vi "example.vi"() -> ()   [LabVIEW 2020]
uses:
  g_industrial_cam/Device Enumeration.ctl
  g_industrial_cam/Camera/Camera.lvclass/Camera.ctl
  g_industrial_cam/Buffer/Buffer.lvclass/Buffer.ctl
  g_industrial_cam/Camera/GetSetPixelFormat.vi
  g_industrial_cam/Buffer/Create from Handle.vi
  g_industrial_cam/Camera/Check Not Disconnected.vi
  <vilib>/Utility/error.llb/Error Cluster From Error Code.vi
  g_industrial_cam/Buffer/Buffer.lvclass
  g_industrial_cam/Camera/Camera.lvclass
panel:
  out "error out":errorcluster
  out "Image":T1(plugin-control)
  out "Devices":T2[](array[typedef])
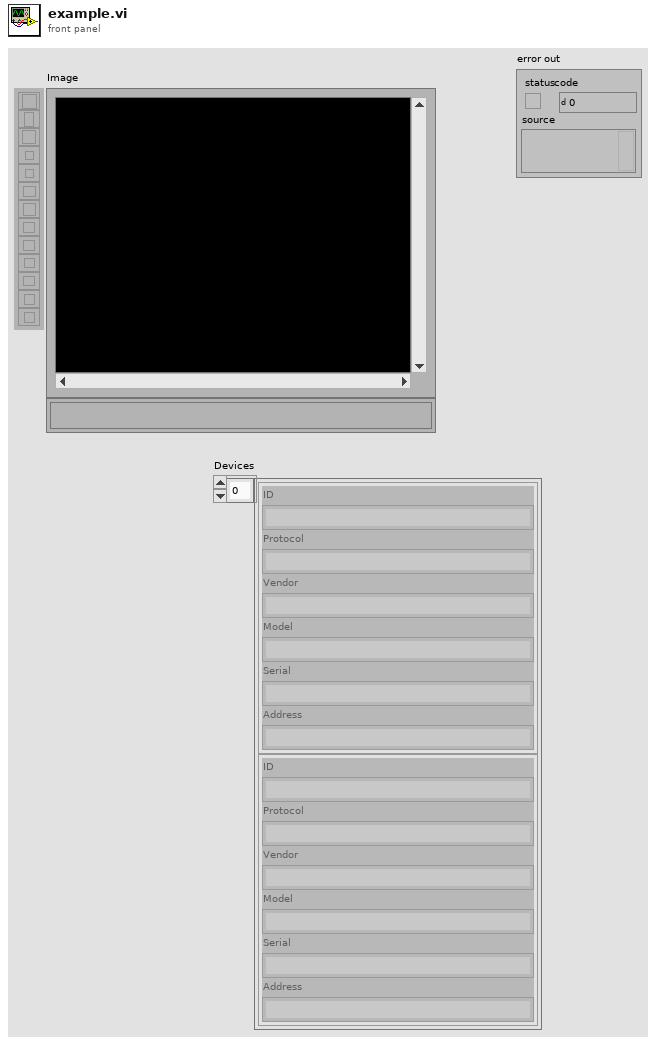
[diagram p1: front panel]
types:
  T1 = typedef "IMAQ Image.ctl" = refnum<image>
  T2 = typedef "Device Enumeration.ctl" = cluster{"ID":string, "Protocol":string, "Vendor":string, "Model":string, "Serial":string, "Address":string}
  T3 = typedef "Image Type" = u32
  T4 = typedef "Buffer.lvclass/Image Size.ctl" = cluster{"Width":u16, "Height":u16}
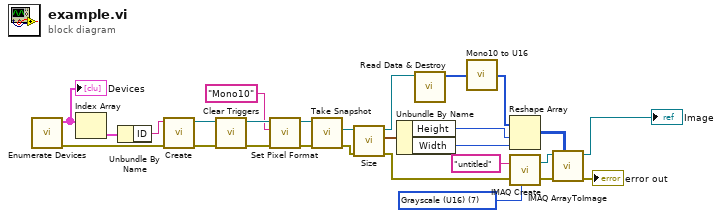
[diagram p0: block diagram]
diagram:
  w27 = T3 7 items=["Grayscale (U8)", "Grayscale (I16)", "Grayscale (SGL)", "Complex (CSG)", "RGB (U32)", "HSL (U32)", "RGB (U64)", "Grayscale (U16)"] ("Image Type")
  n1 = call "Enumerate Devices.vi"() -> ("error out"=w24:errorcluster, "Devices"=w26:T2[])  [unwired: 10 in]
  "Devices" <- w26
  n2 = Index Array(array=w26) -> (element=w25:T2)  [unwired: 1 in]
  n3 = Unbundle By Name(w25) -> ("ID"=w23:string)
  n4 = call "Create.vi"("error in (no error)"=w24, "Identifier (ID, IP etc)"=w23) -> ("error out"=w22:errorcluster, "Camera"=w21:refnum<class "Camera.lvclass">)  [unwired: 8 in]
  n5 = call "Clear Triggers.vi"("error in (no error)"=w22, "Camera in"=w21) -> ("error out"=w20:errorcluster, "Camera"=w19:refnum<class "Camera.lvclass">)  [unwired: 8 in]
  n6 = call "Set Pixel Format.vi"("error in (no error)"=w20, "Pixel Format"="Mono10", "Camera in"=w19) -> ("error out"=w17:errorcluster, "Camera"=w16:refnum<class "Camera.lvclass">)  [unwired: 7 in]
  n7 = call "Take Snapshot.vi"("error in (no error)"=w17, "Camera in"=w16) -> ("error out"=w3:errorcluster, "New Buffer"=w11:refnum<class "Buffer.lvclass">)  [unwired: 7 in, 1 out]
  n8 = call "Size.vi"("error in (no error)"=w3, "Buffer Data in"=w11) -> ("error out"=w2:errorcluster, "Image Size"=w8:T4, "Buffer Data"=w10:refnum<class "Buffer.lvclass">)  [unwired: 7 in]
  n9 = Unbundle By Name(w8) -> ("Height"=w7:u16, "Width"=w6:u16)
  n10 = call "Read Data & Destroy.vi"("Buffer in"=w10) -> ("Data"=w15:u8[])  [unwired: 9 in, 1 out]
  n11 = call "Mono10 to U16.vi"("Mono 10 Data"=w15) -> ("U16 Pixels"=w13:u16[])
  n12 = Reshape Array(w13, w7, w6) -> (w12:u16[][])
  n13 = call "IMAQ Create"("Image Name"="untitled", "Image Type"=w27, "error in (no error)"=w2) -> ("New Image"=w14:T1, "error out"=w9:errorcluster)  [unwired: 2 in]
  n14 = call "IMAQ ArrayToImage"("Image Pixels (U16)"=w12, "error in (no error)"=w9, "Image"=w14) -> ("error out"=→"error out":errorcluster, "Image Out"=→"Image":T1)  [unwired: 7 in]
